vi "DDE Open Conversation.vi"(6 "error in (no error)":errorcluster, 8 "topic":string, 9 "service":string) -> (0 "error out":errorcluster, 3 "conversation refnum":u32)   [LabVIEW 2010]
doc: "Establishes a connection between LabVIEW and another application. You must call this VI before you use any other DDE VIs (except Server VIs). Refer to the Using DDE in LabVIEW Application Note for more information about DDE.\n\n<B>service</B> is the name of the DDE server.\n\n<B>topic</B> is the name of the DDE topic.\n\n<B>error in</B> describes error conditions that occur before this VI or function runs. The default is no error. If an error occurred before this VI or function runs, the VI or function passes the <B>error in</B> value to <B>error out</B>. This VI or function runs normally only if no error occurs before this VI or function runs. If an error occurs while this VI or function runs, it runs normally and sets its own error status in <B>error out</B>. Use the Simple Error Handler or General Error Handler VIs to display the description of the error code. Use <B>error in</B> and <B>error out</B> to check errors and to specify execution order by wiring <B>error out</B> from one node to <B>error in</B> of the next node.\n\n<B>status</B> is TRUE (X) if an error occurred before this VI or function ran or FALSE (checkmark) to indicate a warning or that no error occurred before this VI or function ran. The default is FALSE.\n\n<B>code</B> is the error or warning code. The default is 0. If <B>status</B> is TRUE, <B>code</B> is a non-zero error code. If <B>status</B> is FALSE, <B>code</B> is 0 or a warning code.\n\n<B>source</B> describes the origin of the error or warning and is, in most cases, the name of the VI or function that produced the error or warning. The default is an empty string.\n\n<B>conversation refnum</B> is a refnum that uniquely identifies this DDE conversation. If an error occurs, the value is 0.\n\n<B>error out</B> contains error information. If <B>error in</B> indicates that an error occurred before this VI or function ran, <B>error out</B> contains the same error information. Otherwise, it describes the error status that this VI or function produces. Right-click the <B>error out</B> indicator on the front panel and select <B>Explain Error</B> from the shortcut menu for more information about the error.\n\n<B>status</B> is TRUE (X) if an error occurred or FALSE (checkmark) to indicate a warning or that no error occurred.\n\n<B>code</B> is the error or warning code. If <B>status</B> is TRUE, <B>code</B> is a non-zero error code. If <B>status</B> is FALSE, <B>code</B> is 0 or a warning code.\n\n<B>source</B> describes the origin of the error or warning and is, in most cases, the name of the VI or function that produced the error or warning.\n\n\n\nEstablishes a connection between LabVIEW and another application. You must call this VI before you use any other DDE VIs (except Server VIs). Refer to the Using DDE in LabVIEW Application Note for more information about DDE.\n\n<B>service</B> is the name of the DDE server.\n\n<B>topic</B> is the name of the DDE topic.\n\n<B>error in</B> describes error conditions that occur before this VI or function runs. The default is no error. If an error occurred before this VI or function runs, the VI or function passes the <B>error in</B> value to <B>error out</B>. This VI or function runs normally only if no error occurs before this VI or function runs. If an error occurs while this VI or function runs, it runs normally and sets its own error status in <B>error out</B>. Use the Simple Error Handler or General Error Handler VIs to display the description of the error code. Use <B>error in</B> and <B>error out</B> to check errors and to specify execution order by wiring <B>error out</B> from one node to <B>error in</B> of the next node.\n\n<B>status</B> is TRUE (X) if an error occurred before this VI or function ran or FALSE (checkmark) to indicate a warning or that no error occurred before this VI or function ran. The default is FALSE.\n\n<B>code</B> is the error or warning code. The default is 0. If <B>status</B> is TRUE, <B>code</B> is a non-zero error code. If <B>status</B> is FALSE, <B>code</B> is 0 or a warning code.\n\n<B>source</B> describes the origin of the error or warning and is, in most cases, the name of the VI or function that produced the error or warning. The default is an empty string.\n\n<B>conversation refnum</B> is a refnum that uniquely identifies this DDE conversation. If an error occurs, the value is 0.\n\n<B>error out</B> contains error information. If <B>error in</B> indicates that an error occurred before this VI or function ran, <B>error out</B> contains the same error information. Otherwise, it describes the error status that this VI or function produces. Right-click the <B>error out</B> indicator on the front panel and select <B>Explain Error</B> from the shortcut menu for more information about the error.\n\n<B>status</B> is TRUE (X) if an error occurred or FALSE (checkmark) to indicate a warning or that no error occurred.\n\n<B>code</B> is the error or warning code. If <B>status</B> is TRUE, <B>code</B> is a non-zero error code. If <B>status</B> is FALSE, <B>code</B> is 0 or a warning code.\n\nEstablishes a connection between LabVIEW and another application. You must call this VI before you use any other DDE VIs (except Server VIs). Refer to the Using DDE in LabVIEW Application Note for more information about DDE.\n\n<B>service</B> is the name of the DDE server.\n\n<B>topic</B> is the name of the DDE topic.\n\n<B>error in</B> describes error conditions that occur before this VI or function runs. The default is no error. If an error occurred before this VI or function runs, the VI or function passes the <B>error in</B> value to <B>error out</B>. This VI or function runs normally only if no error occurs before this VI or function runs. If an error occurs while this VI or function runs, it runs normally and sets its own error status in <B>error out</B>. Use the Simple Error Handler or General Error Handler VIs to display the description of the error code. Use <B>error in</B> and <B>error out</B> to check errors and to specify execution order by wiring <B>error out</B> from one node to <B>error in</B> of the next node.\n\n<B>status</B> is TRUE (X) if an error occurred before this VI or function ran or FALSE (checkmark) to indicate a warning or that no error occurred before this VI or function ran. The default is FALSE.\n\n<B>code</B> is the error or warning code. The default is 0. If <B>status</B> is TRUE, <B>code</B> is a non-zero error code. If <B>status</B> is FALSE, <B>code</B> is 0 or a warning code.\n\n<B>source</B> describes the origin of the error or warning and is, in most cases, the name of the VI or function that produced the error or warning. The default is an empty string.\n\n<B>conversation refnum</B> is a refnum that uniquely identifies this DDE conversation. If an error occurs, the value is 0.\n\n<B>error out</B> contains error information. If <B>error in</B> indicates that an error occurred before this VI or function ran, <B>error out</B> contains the same error information. Otherwise, it describes the error status that this VI or function produces. Right-click the <B>error out</B> indicator on the front panel and select <B>Explain Error</B> from the shortcut menu for more information about the error.\n\n<B>status</B> is TRUE (X) if an error occurred or FALSE (checkmark) to indicate a warning or that no error occurred.\n\n<B>code</B> is the error or warning code. If <B>status</B> is TRUE, <B>code</B> is a non-zero error code. If <B>status</B> is FALSE, <B>code</B> is 0 or a warning code.\n\n<B>source</B> describes the origin of the error or warning and is, in most cases, the name of the VI or function that produced the error or warning."
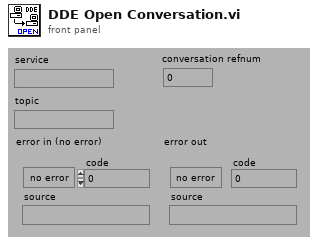
[diagram p1: front panel]
types:
  T1 = cluster{i8, u32[], "service":string, "topic":string, bool}
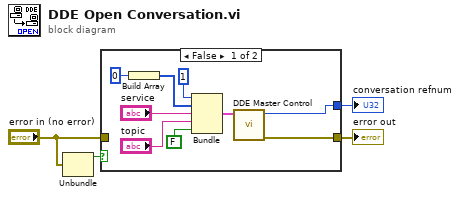
[diagram p0: block diagram]
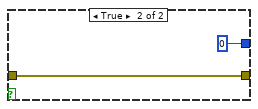
[diagram p2: hidden frame]
diagram:
  n1 = Unbundle("error in (no error)") -> ("status"=w3:bool)  [unwired: 2 out]
  n2 = case shown="False" w3 {
    tunnel: [w7 w15] -> w1
    tunnel: [w12 u32 0] -> w4
    tunnel: "error in (no error)" -> [_ w15]
    frame False {
      n3 = Build Array(u32 0) -> (w5:u32[])
      n4 = Bundle(i8 1, w5, "service"="service", "topic"="topic", FALSE) -> (w8:T1)  [unwired: 1 in]
      n5 = call <vilib>:"DDE Master Control.vi"("input"=w8) -> ("error out"=w7:errorcluster, "refnum"=w12:u32)  [unwired: 4 in, 3 out]
    }
    frame True {
    }
  }
  "conversation refnum" <- w4
  "error out" <- w1
